vi "MedSolve.vi"(6 "Conf. Gral.":T1, 7 "VirtualMapping":u16[][](array[numeric]), 8 "error in (no error)":errorcluster, 10 "Array Parsed Expression in":T3[](array[typedef]), 11 "Variable Data in":T2) -> (0 "error out":errorcluster, 1 "Array":sgl[](array[numeric]), 2 "Array Parsed Expression Out":T3[](array[typedef]), 3 "Variable Data Out":T2, 4 "Array Med":sgl[][](array[numeric]))   [LabVIEW 2014, in "MathLoop.lvlib"]
doc: "Calcula solo el valor final de Resultado."
uses:
  MathLoop.lvlib
  TypeDefs/ParsedExpression.ctl
  TypeDefs/typeMed.ctl
  TypeDefs/Conf. Gral.ctl
  <vilib>/Analysis/baseanly.llb/Mean.vi
  <vilib>/Analysis/baseanly.llb/Mean (DBL).vi
  <vilib>/Analysis/2dsp.llb/FFT.vi
  <vilib>/Analysis/2dsp.llb/Real FFT.vi
  <vilib>/Analysis/2dsp.llb/Inverse FFT.vi
  <vilib>/Analysis/2dsp.llb/Inverse Complex FFT.vi
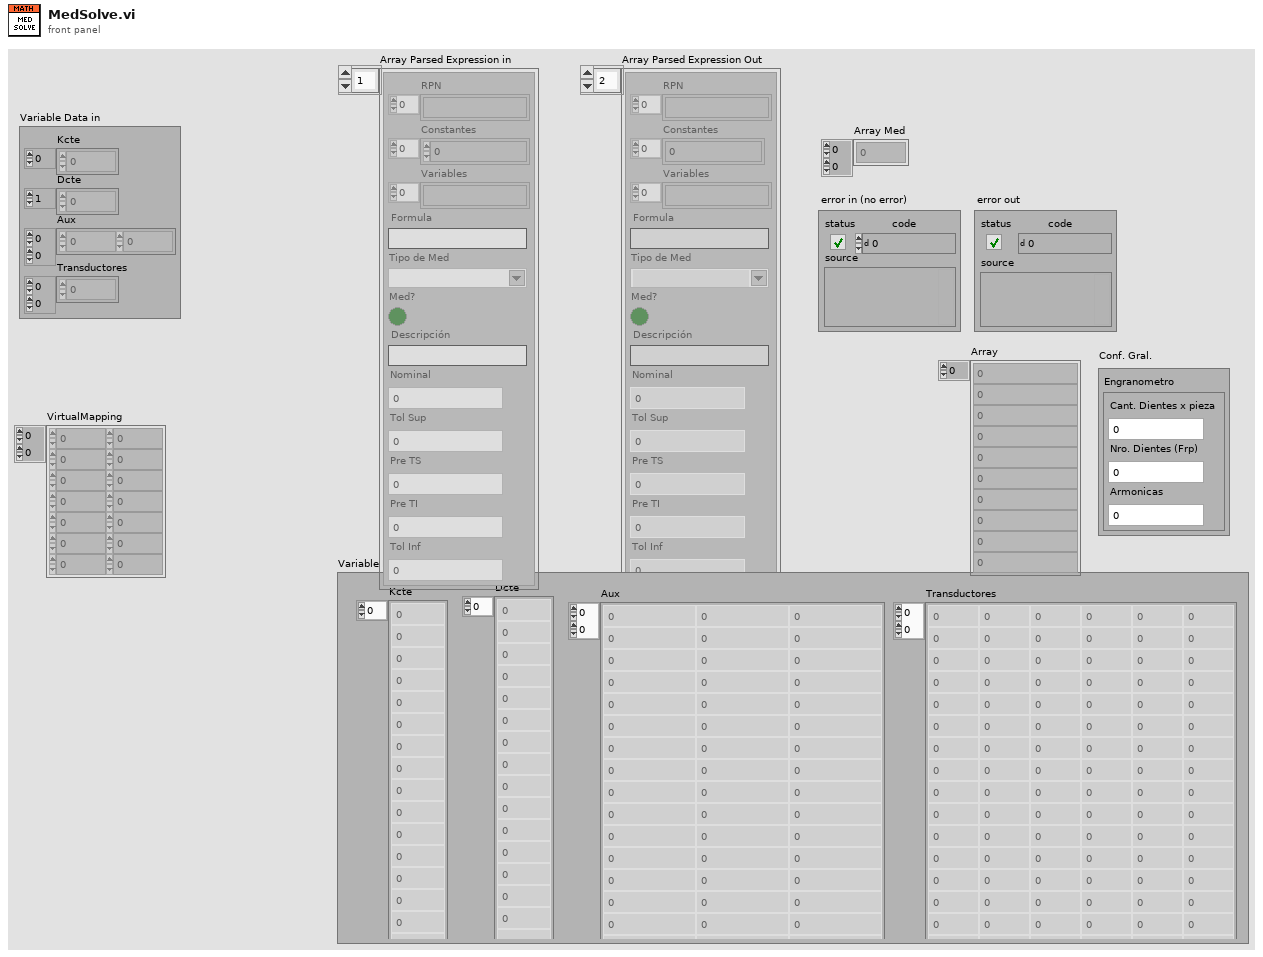
[diagram p1: front panel]
types:
  T1 = typedef "MathLoop.lvlib/Conf. Gral.ctl" = cluster{"Engranometro":cluster{"Cant. Dientes x pieza":i32, "Nro. Dientes (Frp)":i32, "Armonicas":i32}}
  T2 = cluster{"Kcte":sgl[], "Dcte":sgl[], "Aux":sgl[][], "Transductores":sgl[][]}
  T3 = typedef "MathLoop.lvlib/ParsedExpression.ctl" = cluster{"RPN ":string[], "Constantes":sgl[], "Variables":string[], "Formula":string, "Tipo de Med":T4, "Med?":bool, "Descripción":string, "Nominal":sgl, "Tol Sup":sgl, "Pre TS":sgl, "Pre TI":sgl, "Tol Inf":sgl}
  T4 = typedef "MathLoop.lvlib/typeMed.ctl" = string
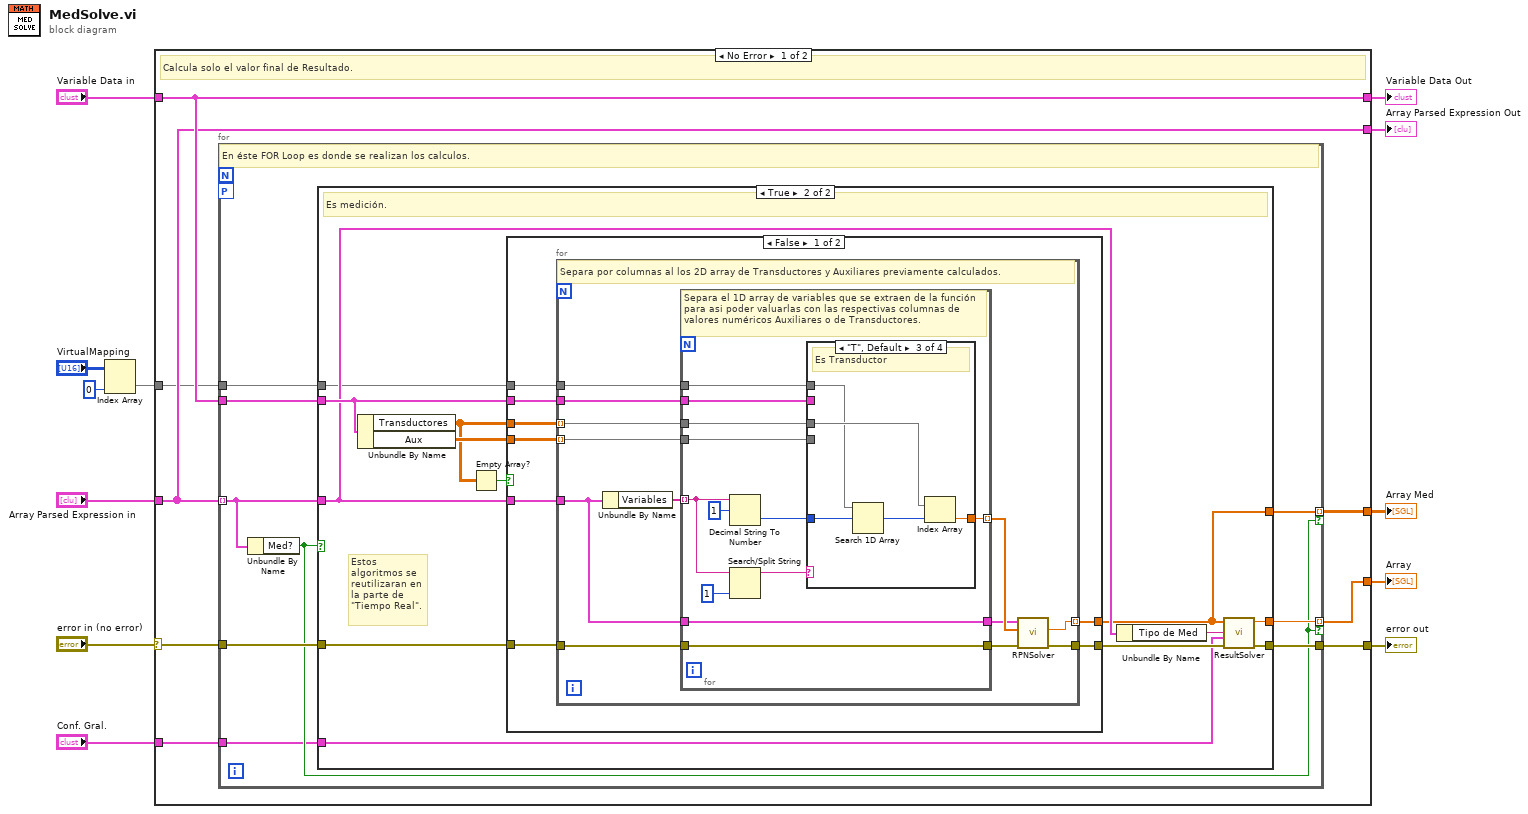
[diagram p0: block diagram]
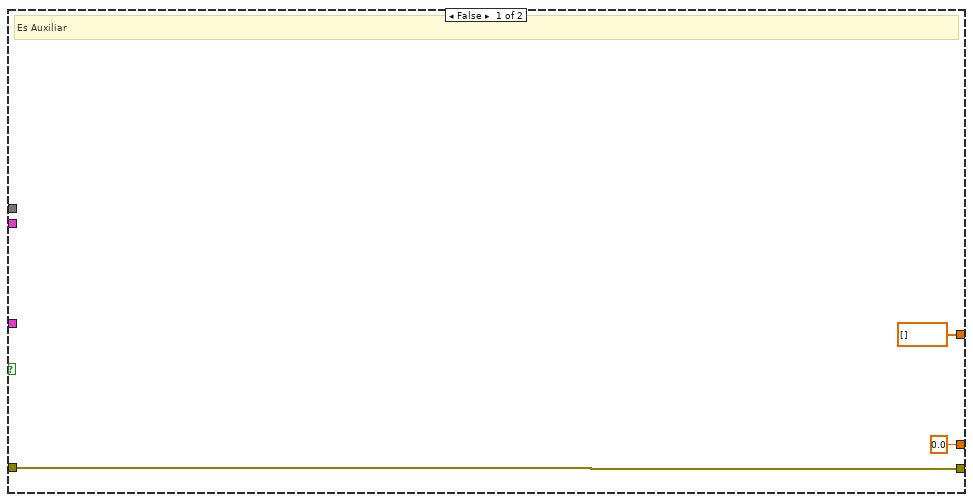
[diagram p2: hidden frame]
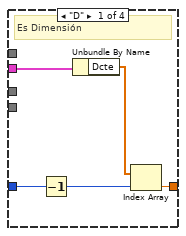
[diagram p3: hidden frame]
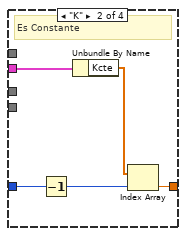
[diagram p4: hidden frame]
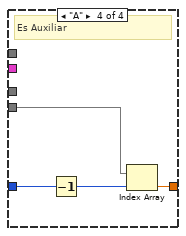
[diagram p5: hidden frame]
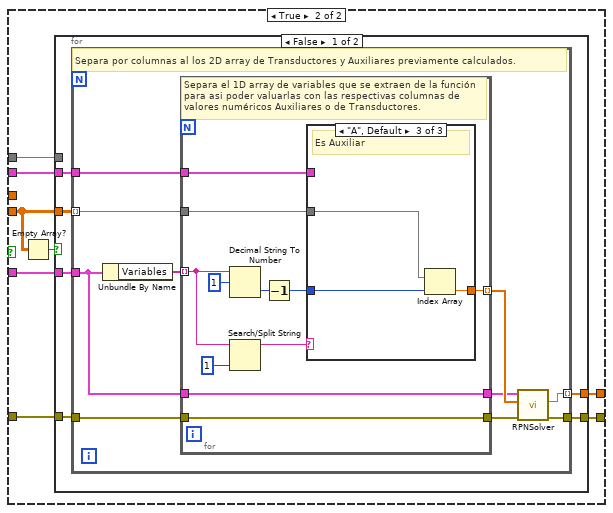
[diagram p6: hidden frame]
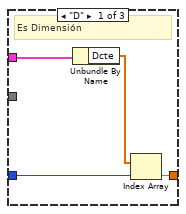
[diagram p7: hidden frame]
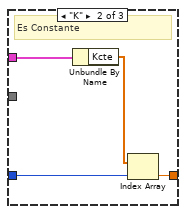
[diagram p8: hidden frame]
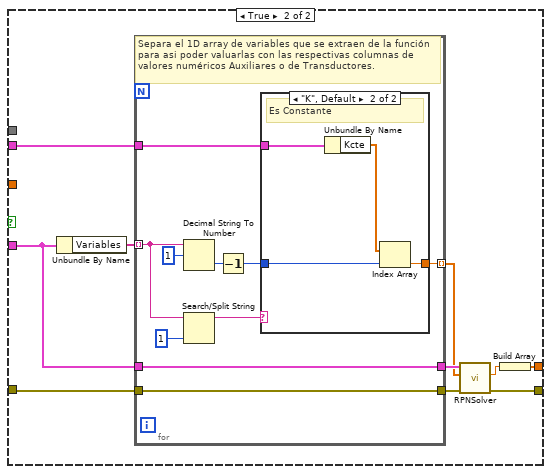
[diagram p9: hidden frame]
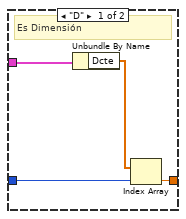
[diagram p10: hidden frame]
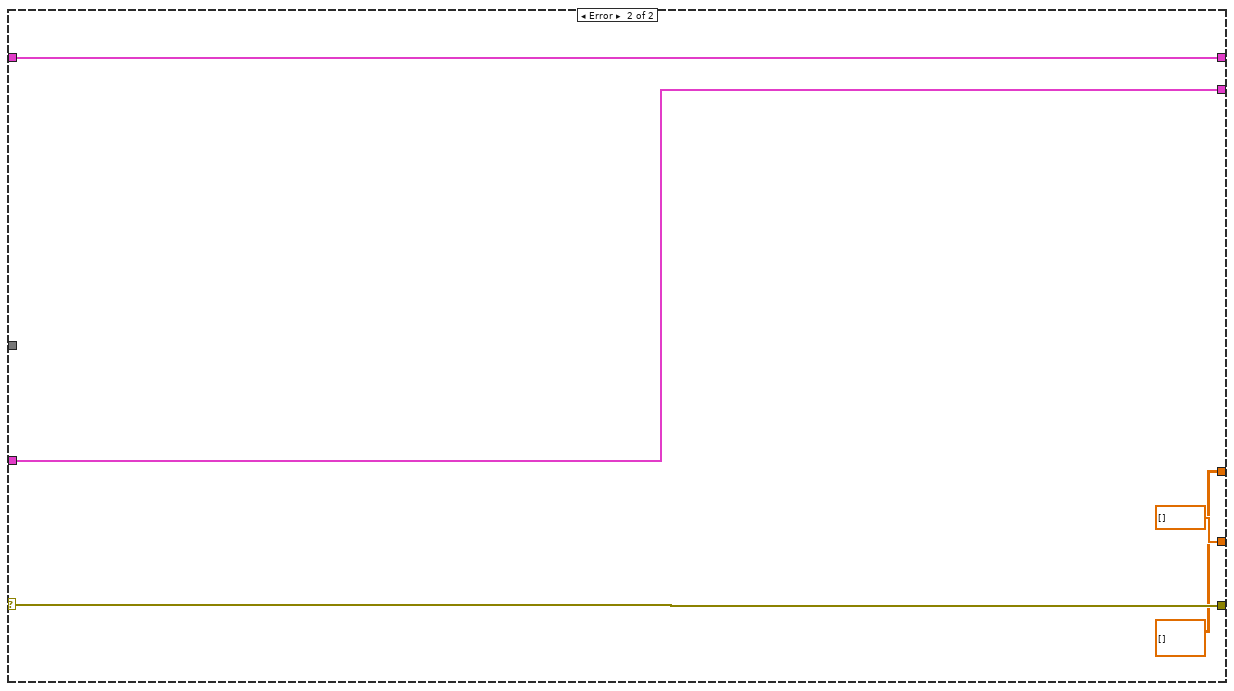
[diagram p11: hidden frame]
diagram:
  n1 = Index Array(array="VirtualMapping", index (col)=0 ("disabled index (col)")) -> (element=w1:u16[])  [unwired: 1 in]
  n2 = case shown="No Error" "error in (no error)" {
    selector: "error in (no error)" -> [w19 w173]
    tunnel: "Variable Data in" -> [w17 w174]
    tunnel: "Array Parsed Expression in" -> [w16 w175]
    tunnel: [w20 w173] -> w10
    tunnel: [w16 w175] -> w9
    tunnel: [w17 w174] -> w8
    tunnel: [w18 sgl[] []] -> w6
    tunnel: [w15 sgl[][] []] -> w5
    tunnel: "Conf. Gral." -> [w14 _]
    tunnel: w1 -> [w13 _]
    frame No Error {
      # "Calcula solo el valor final de Resultado."
      n3 = for {
        tunnel: w16 -> [w23] mode=indexing
        tunnel: w17 -> [w26]
        tunnel: [w29] -> w18 mode=indexing if=w24
        tunnel: [w28] -> w20
        tunnel: w19 -> [w27]
        tunnel: [w25] -> w15 mode=indexing if=w24
        tunnel: w14 -> [w22]
        workers-P: _ -> [_]
        tunnel: w13 -> [w21]
        # "En éste FOR Loop es donde se realizan los calculos."
        n4 = Unbundle By Name(w23) -> ("Med?"=w24:bool)
        n5 = case shown="True" w24 {
          tunnel: w23 -> [_ w42]
          tunnel: [sgl 0.0 ("Result") w43] -> w29
          tunnel: [w32 w38] -> w28
          tunnel: w27 -> [w32 w45]
          tunnel: w26 -> [_ w44]
          tunnel: [sgl[] [] w39] -> w25
          tunnel: w22 -> [_ w36]
          tunnel: w21 -> [_ w33]
          frame False {
            # "Es Auxiliar"
          }
          frame True {
            # "Estos algoritmos se reutilizaran en la parte de \"Tiempo Real\"."
            # "Es medición."
            n6 = Unbundle By Name(w44) -> ("Transductores"=w34:sgl[][], "Aux"=w40:sgl[][])
            n7 = Empty Array?(array=w34) -> (empty?=w35:bool)
            n8 = case shown="False" w35 {
              tunnel: w45 -> [w53 w102]
              tunnel: w44 -> [w52 w104]
              tunnel: w42 -> [w51 w103]
              tunnel: w34 -> [w50 _]
              tunnel: w40 -> [w49 w98]
              tunnel: [w48 w100] -> w39
              tunnel: [w47 w101] -> w37
              tunnel: w33 -> [w46 w97]
              frame False {
                n9 = for {
                  tunnel: [w60] -> w48 mode=indexing
                  tunnel: w51 -> [w64]
                  tunnel: w52 -> [w61]
                  tunnel: w50 -> [w62] mode=indexing
                  tunnel: w53 -> [w63]
                  tunnel: w49 -> [w59] mode=indexing
                  tunnel: [w58] -> w47
                  tunnel: w46 -> [w54]
                  # "Separa por columnas al los 2D array de Transductores y Auxiliares previamente calculados."
                  n10 = Unbundle By Name(w64) -> ("Variables"=w65:string[])
                  n11 = for {
                    tunnel: w65 -> [w70] mode=indexing
                    tunnel: w64 -> [w75]
                    tunnel: w63 -> [w73]
                    tunnel: w62 -> [w77]
                    tunnel: w61 -> [w76]
                    tunnel: [w75] -> w55
                    tunnel: [w74] -> w56 mode=indexing
                    tunnel: [w73] -> w57
                    tunnel: w59 -> [w72]
                    tunnel: w54 -> [w67]
                    # "Separa el 1D array de variables que se extraen de la función para asi poder valuarlas con las respectivas columnas de valores numéricos Auxiliares o de Transductores."
                    n12 = Decimal String To Number(string=w70, offset=1) -> (number=w66:i32)  [unwired: 1 in, 1 out]
                    n13 = Search/Split String(string=w70, offset (0)=1) -> (substring before match=w68:string)  [unwired: 1 in, 2 out]
                    n14 = case shown="\"T\", Default" w68 {
                      tunnel: [w80 w87 w92 w96] -> w74
                      tunnel: w77 -> [_ _ w91 _]
                      tunnel: w76 -> [w81 w86 _ _]
                      tunnel: w72 -> [_ _ _ w95]
                      tunnel: w66 -> [w79 w84 w88 w94]
                      tunnel: w67 -> [_ _ w90 _]
                      frame "D" {
                        # "Es Dimensión"
                        n15 = Decrement(x=w79) -> (x-1=w78:i32)
                        n16 = Unbundle By Name(w81) -> ("Dcte"=w82:sgl[])
                        n17 = Index Array(array=w82, index=w78) -> (element=w80:sgl)
                      }
                      frame "K" {
                        # "Es Constante"
                        n18 = Decrement(x=w84) -> (x-1=w83:i32)
                        n19 = Unbundle By Name(w86) -> ("Kcte"=w85:sgl[])
                        n20 = Index Array(array=w85, index=w83) -> (element=w87:sgl)
                      }
                      frame "T", Default {
                        # "Es Transductor"
                        n21 = Search 1D Array(1D array=w90, element=w88) -> (index of element=w89:i32)  [unwired: 1 in]
                        n22 = Index Array(array=w91, index=w89) -> (element=w92:sgl)
                      }
                      frame "A" {
                        # "Es Auxiliar"
                        n23 = Decrement(x=w94) -> (x-1=w93:i32)
                        n24 = Index Array(array=w95, index=w93) -> (element=w96:sgl)
                      }
                    }
                  }
                  n25 = call "RPNSolver.vi"("error in"=w57, "Variable Value Array"=w56, "Parsed Expression In"=w55) -> ("error out"=w58:errorcluster, "Numeric"=w60:sgl)  [unwired: 5 in, 1 out]
                }
              }
              frame True {
                n26 = Empty Array?(array=w98) -> (empty?=w99:bool)
                n27 = case shown="False" w99 {
                  tunnel: w104 -> [w110 w147]
                  tunnel: w98 -> [w109 _]
                  tunnel: w103 -> [w108 w145]
                  tunnel: w102 -> [w107 w146]
                  tunnel: [w106 w148] -> w101
                  tunnel: [w105 w143] -> w100
                  tunnel: w97 -> [_ _]
                  frame False {
                    n28 = for {
                      tunnel: [w116] -> w105 mode=indexing
                      tunnel: w108 -> [w119]
                      tunnel: w110 -> [w117]
                      tunnel: w107 -> [w118]
                      tunnel: w109 -> [w115] mode=indexing
                      tunnel: [w114] -> w106
                      # "Separa por columnas al los 2D array de Transductores y Auxiliares previamente calculados."
                      n29 = Unbundle By Name(w119) -> ("Variables"=w120:string[])
                      n30 = for {
                        tunnel: w120 -> [w123] mode=indexing
                        tunnel: w119 -> [w130]
                        tunnel: w118 -> [w128]
                        tunnel: w117 -> [w131]
                        tunnel: [w130] -> w111
                        tunnel: [w129] -> w112 mode=indexing
                        tunnel: [w128] -> w113
                        tunnel: w115 -> [w127]
                        # "Separa el 1D array de variables que se extraen de la función para asi poder valuarlas con las respectivas columnas de valores numéricos Auxiliares o de Transductores."
                        n31 = Decimal String To Number(string=w123, offset=1) -> (number=w126:i32)  [unwired: 1 in, 1 out]
                        n32 = Search/Split String(string=w123, offset (0)=1) -> (substring before match=w121:string)  [unwired: 1 in, 2 out]
                        n33 = Decrement(x=w126) -> (x-1=w124:i32)
                        n34 = case shown="\"A\", Default" w121 {
                          tunnel: [w133 w139 w142] -> w129
                          tunnel: w131 -> [w134 w138 _]
                          tunnel: w127 -> [_ _ w141]
                          tunnel: w124 -> [w132 w136 w140]
                          frame "D" {
                            # "Es Dimensión"
                            n35 = Unbundle By Name(w134) -> ("Dcte"=w135:sgl[])
                            n36 = Index Array(array=w135, index=w132) -> (element=w133:sgl)
                          }
                          frame "K" {
                            # "Es Constante"
                            n37 = Unbundle By Name(w138) -> ("Kcte"=w137:sgl[])
                            n38 = Index Array(array=w137, index=w136) -> (element=w139:sgl)
                          }
                          frame "A", Default {
                            # "Es Auxiliar"
                            n39 = Index Array(array=w141, index=w140) -> (element=w142:sgl)
                          }
                        }
                      }
                      n40 = call "RPNSolver.vi"("error in"=w113, "Variable Value Array"=w112, "Parsed Expression In"=w111) -> ("error out"=w114:errorcluster, "Numeric"=w116:sgl)  [unwired: 5 in, 1 out]
                    }
                  }
                  frame True {
                    n41 = Unbundle By Name(w145) -> ("Variables"=w149:string[])
                    n42 = for {
                      tunnel: w149 -> [w155] mode=indexing
                      tunnel: w145 -> [w161]
                      tunnel: w146 -> [w159]
                      tunnel: w147 -> [w162]
                      tunnel: [w161] -> w152
                      tunnel: [w160] -> w151 mode=indexing
                      tunnel: [w159] -> w150
                      # "Separa el 1D array de variables que se extraen de la función para asi poder valuarlas con las respectivas columnas de valores numéricos Auxiliares o de Transductores."
                      n43 = Decimal String To Number(string=w155, offset=1) -> (number=w158:i32)  [unwired: 1 in, 1 out]
                      n44 = Search/Split String(string=w155, offset (0)=1) -> (substring before match=w153:string)  [unwired: 1 in, 2 out]
                      n45 = Decrement(x=w158) -> (x-1=w156:i32)
                      n46 = case shown="\"K\", Default" w153 {
                        tunnel: [w164 w170] -> w160
                        tunnel: w162 -> [w165 w169]
                        tunnel: w156 -> [w163 w167]
                        frame "D" {
                          # "Es Dimensión"
                          n47 = Unbundle By Name(w165) -> ("Dcte"=w166:sgl[])
                          n48 = Index Array(array=w166, index=w163) -> (element=w164:sgl)
                        }
                        frame "K", Default {
                          # "Es Constante"
                          n49 = Unbundle By Name(w169) -> ("Kcte"=w168:sgl[])
                          n50 = Index Array(array=w168, index=w167) -> (element=w170:sgl)
                        }
                      }
                    }
                    n51 = call "RPNSolver.vi"("error in"=w150, "Variable Value Array"=w151, "Parsed Expression In"=w152) -> ("error out"=w148:errorcluster, "Numeric"=w144:sgl)  [unwired: 5 in, 1 out]
                    n52 = Build Array(w144) -> (w143:sgl[])
                  }
                }
              }
            }
            n53 = Unbundle By Name(w42) -> ("Tipo de Med"=w41:T4)
            n54 = call "ResultSolver.vi"("error in (no error)"=w37, "Conf. Gral."=w36, "Tipo de Med"=w41, "Array"=w39) -> ("error out"=w38:errorcluster, "Result"=w43:sgl)  [unwired: 6 in]
          }
        }
      }
    }
    frame Error {
    }
  }
  "error out" <- w10
  "Array Parsed Expression Out" <- w9
  "Variable Data Out" <- w8
  "Array" <- w6
  "Array Med" <- w5
